vi "外观 1.vi"(0 "Data In":T5 caption="数据输入", 2 "Display State In":T3 caption="显示状态输入", 3 "Container State":T4 caption="容器状态") -> (6 "Data Out":T5 caption="数据输出", 7 "Display State Out":T3 caption="显示状态输出", 8 "Action":T2 caption="动作")   [LabVIEW 2016, in "曲线模型.xctl"]
uses:
  <vilib>/_xctls/Container State.ctl
  <vilib>/_xctls/Action.ctl
  <vilib>/_xctls/XControlSupport.lvlib
  <vilib>/Utility/config.llb/NI_LVConfig.lvlib
panel:
  in  "曲线模型":T1={"标液浓度1"=0.0, "样品1 F0"=0.0, "样品1 F1"=0.0, "测量吸光度1"=0.0, "样品1启用"=FALSE, "标液浓度2"=0.0, "样品2 F0"=0.0, "样品2 F1"=0.0, "测量吸光度2"=0.0, "样品2启用"=FALSE, "标液浓度3"=0.0, "样品3 F0"=0.0, "样品3 F1"=0.0, "测量吸光度3"=0.0, "样品3启用"=FALSE, "标液浓度4"=0.0, "样品4 F0"=0.0, "样品4 F1"=0.0, "测量吸光度4"=0.0, "样品4启用"=FALSE, "标液浓度5"=0.0, "样品5 F0"=0.0, "样品5 F1"=0.0, "测量吸光度5"=0.0, "样品5启用"=FALSE, "模型"=enum."线性", "method"=enum."最小二乘", "精度"=4.0, "XY图"=[], "拟合公式"="", "r^2"=0.0, "吸光值算法"=enum."对数"} {"r^2" format="%.7g"}
  # "标液浓度"
  # "F0"
  # "F1"
  # "吸光值显示"
  # "辅\n助\n计\n算\n区"
  # "样品一"
  # "样品二"
  # "样品三"
  # "样品四"
  # "样品五"
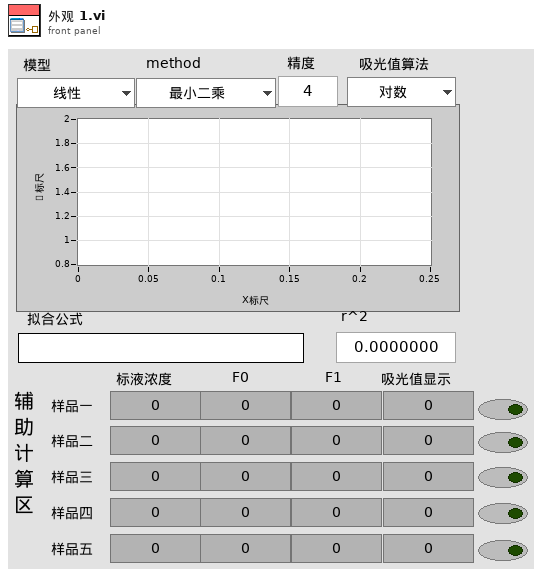
[diagram p1: front panel]
types:
  T1 = typedef "曲线模型.xctl/曲线模型外观.ctl" = cluster{"标液浓度1":dbl, "样品1 F0":dbl, "样品1 F1":dbl, "测量吸光度1":dbl, "样品1启用":bool, "标液浓度2":dbl, "样品2 F0":dbl, "样品2 F1":dbl, "测量吸光度2":dbl, "样品2启用":bool, "标液浓度3":dbl, "样品3 F0":dbl, "样品3 F1":dbl, "测量吸光度3":dbl, "样品3启用":bool, "标液浓度4":dbl, "样品4 F0":dbl, "样品4 F1":dbl, "测量吸光度4":dbl, "样品4启用":bool, "标液浓度5":dbl, "样品5 F0":dbl, "样品5 F1":dbl, "测量吸光度5":dbl, "样品5启用":bool, "模型":enum32{"线性", "多项式"}, "method":enum16{"最小二乘", "最小绝对残差", "Bisquare"}, "精度":dbl, "XY图":cluster{"X Values":dbl[], "Y Values":dbl[]}[], "拟合公式":string, "r^2":dbl, "吸光值算法":enum16{"对数", "减法"}}
  T2 = typedef "XControlSupport.lvlib/Action.ctl" = cluster{"Data Changed?":bool, "State Changed?":bool, "Action Name":string}
  T3 = typedef "曲线模型.xctl/状态 1.ctl" = cluster{"模型选择":cluster{"参数":u8, "测量模式":u8, "量程":u8}, "吸光值":cluster{"Value":dbl, "Value 2":dbl, "Value 3":dbl, "Value 4":dbl, "Value 5":dbl}, "浓度":cluster{"标液浓度1":dbl, "标液浓度2":dbl, "标液浓度3":dbl, "标液浓度4":dbl, "标液浓度5":dbl}}
  T4 = typedef "XControlSupport.lvlib/Container State.ctl" = cluster{"Indicator?":bool, "Run Mode?":bool, " Refnum":refnum<vi>}
  T5 = typedef "曲线模型.xctl/数据 1.ctl" = cluster{"X^2":dbl, "X":dbl, "B":dbl, "r^2":dbl}
  T6 = cluster{"曲线模型":T1, "Polynomial Coefficients":dbl[]}
  T7 = cluster{"Value":dbl, "Value 2":dbl, "Value 3":dbl, "Value 4":dbl, "Value 5":dbl}
  T8 = typedef "NI_LVConfig.lvlib/Config Data RefNum.ctl" = refnum<k1>
  T9 = cluster{"Polynomial Coefficients[0]":dbl, "Polynomial Coefficients[1]":dbl, "Polynomial Coefficients[2]":dbl, "Polynomial Coefficients[3]":dbl}
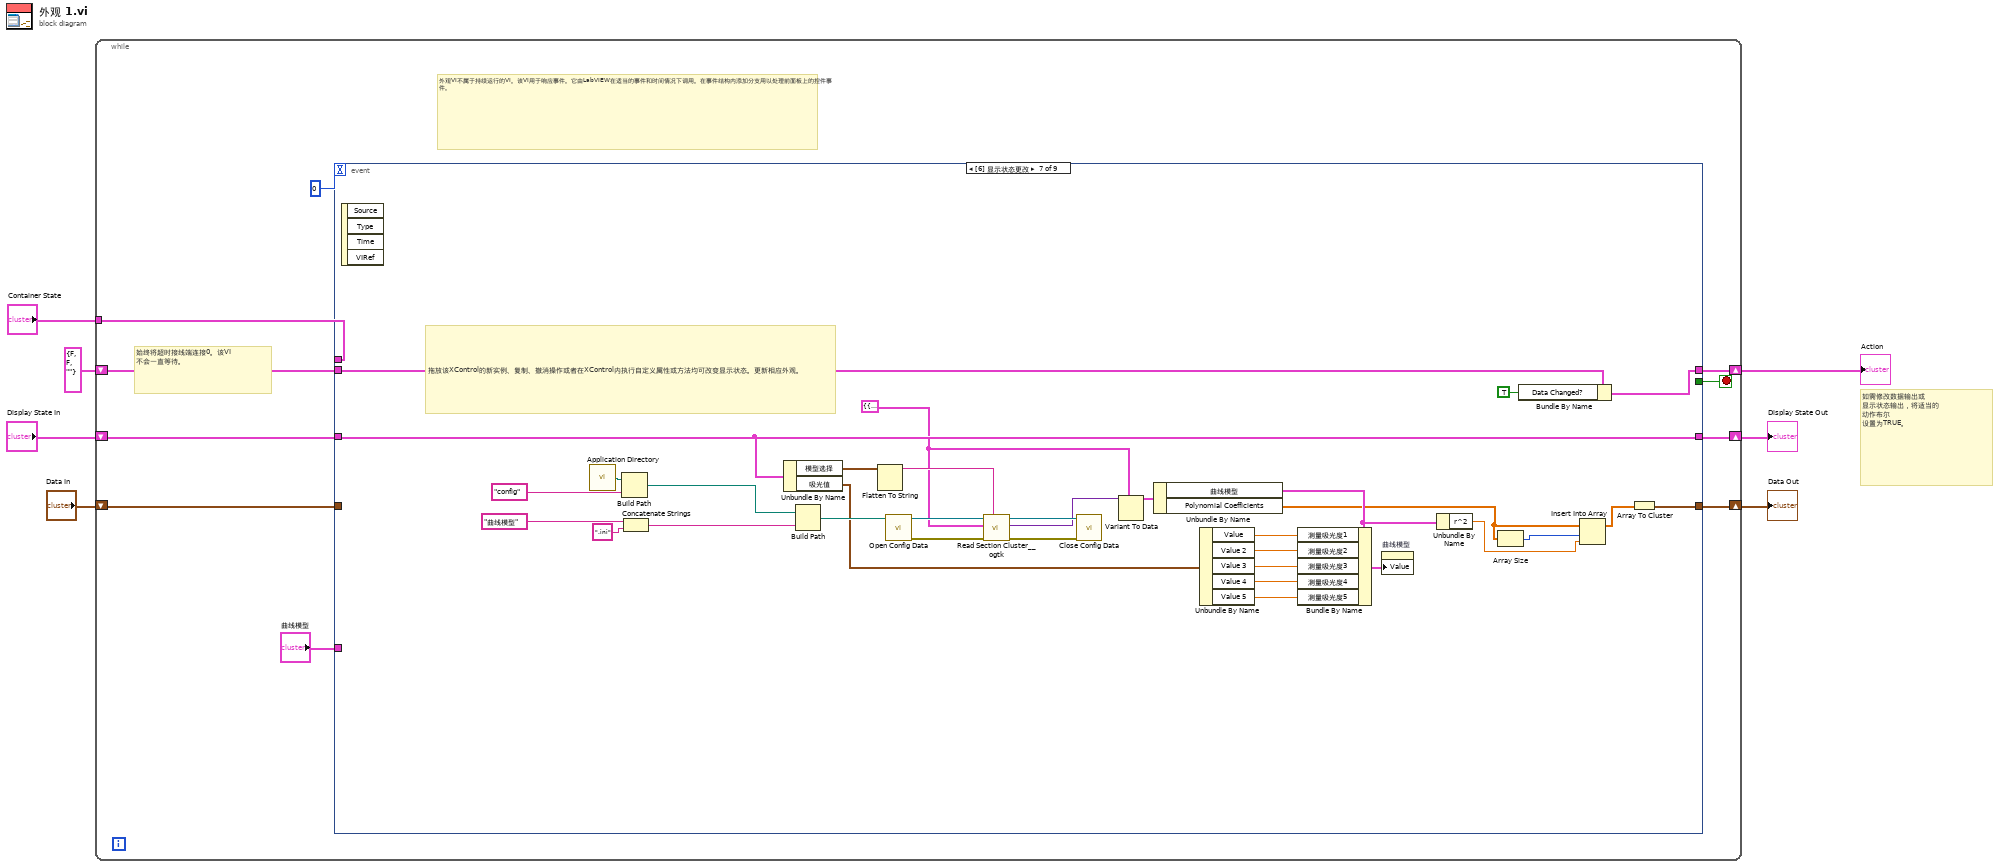
[diagram p0: block diagram]
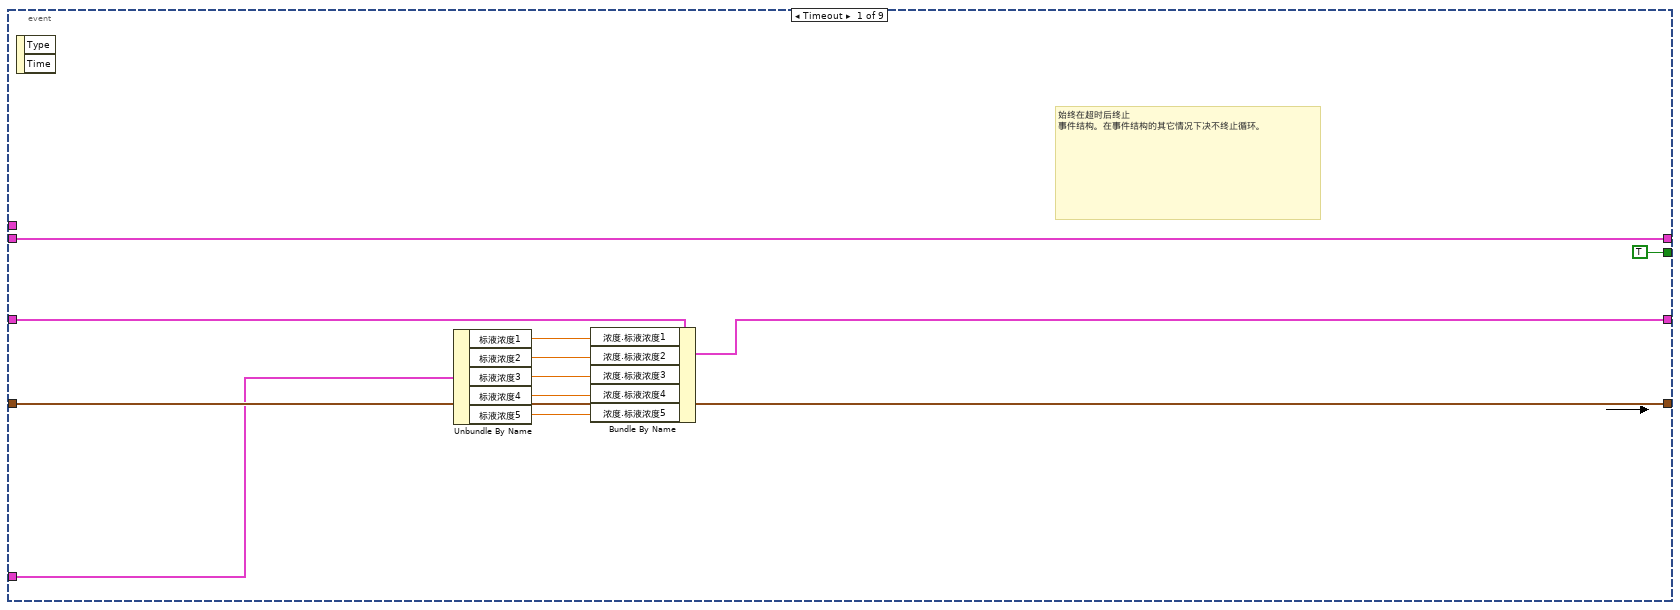
[diagram p2: hidden frame]
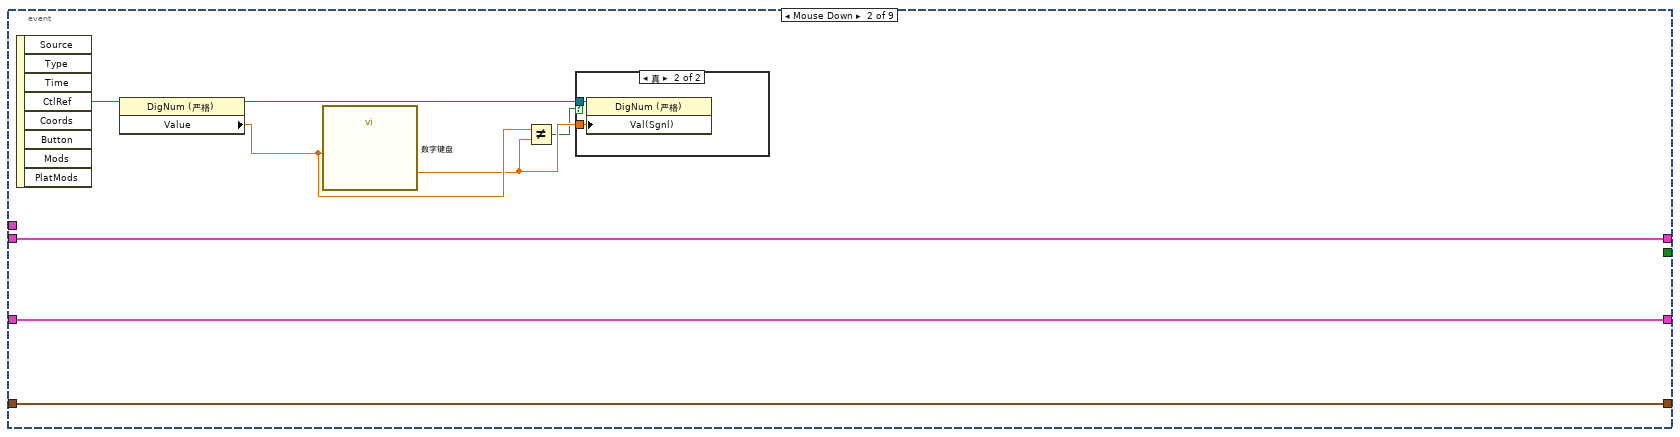
[diagram p3: hidden frame]
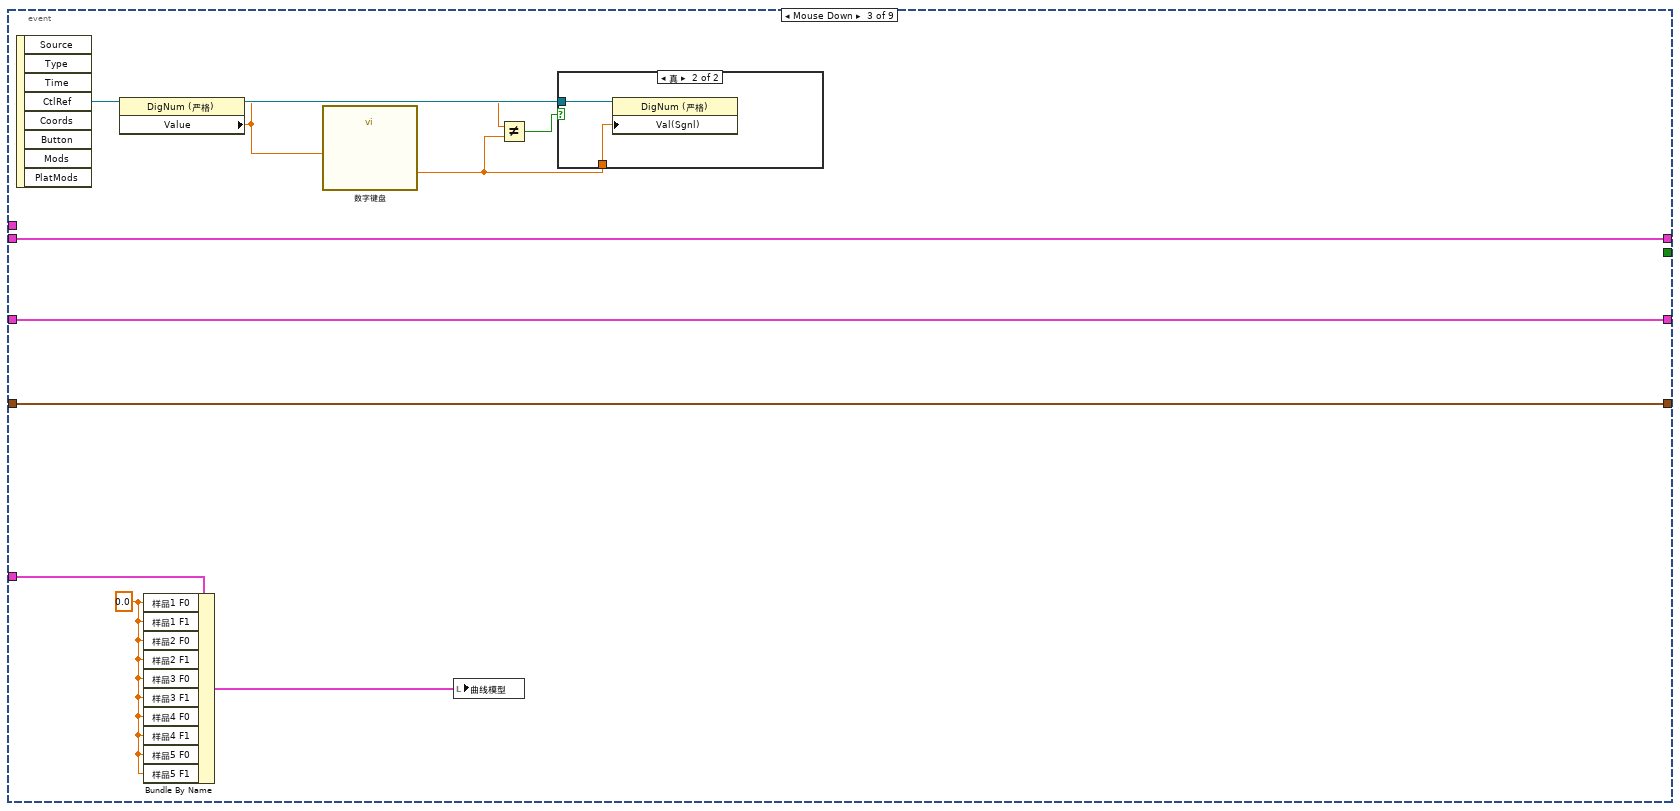
[diagram p5: hidden frame]
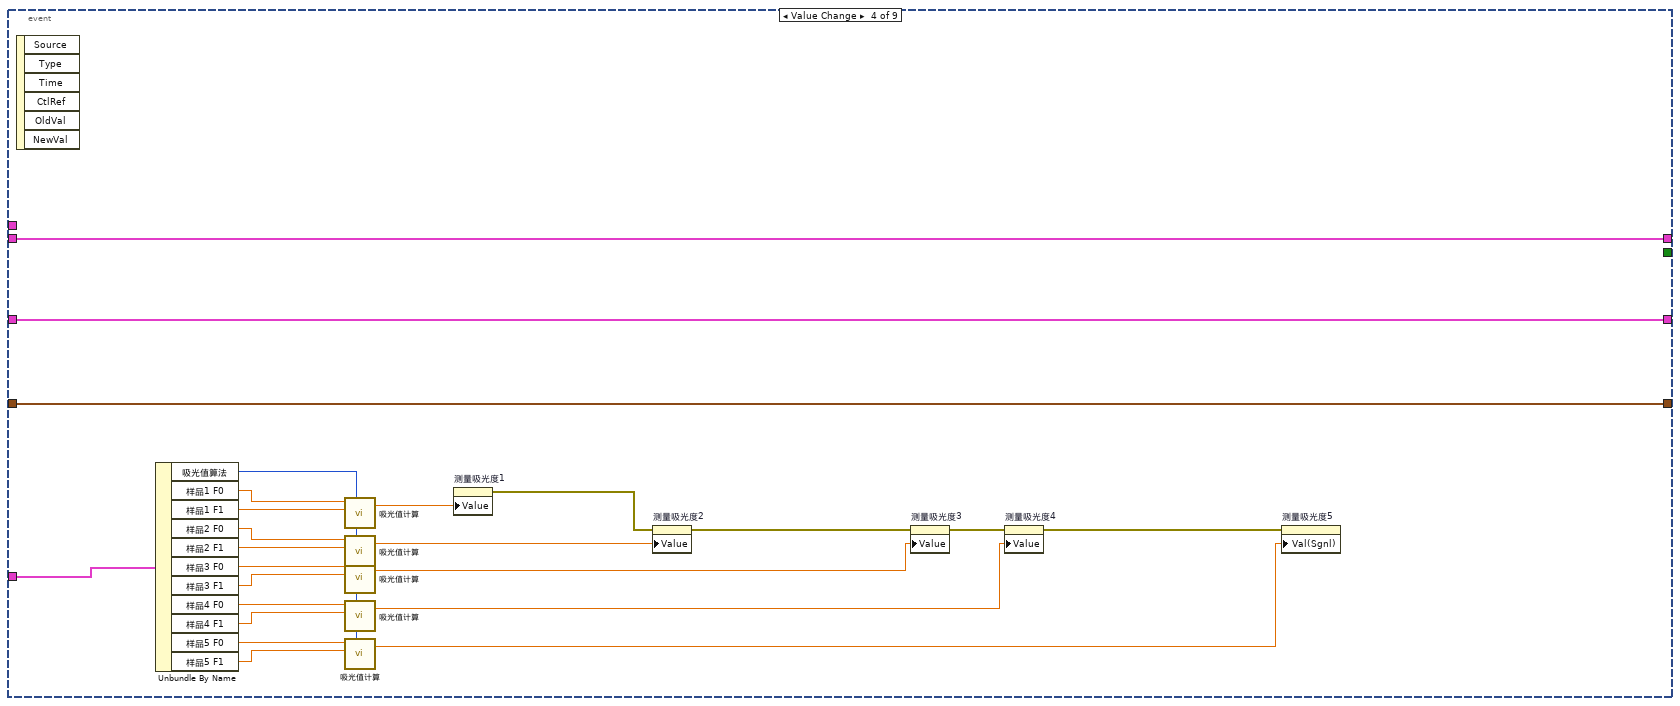
[diagram p7: hidden frame]
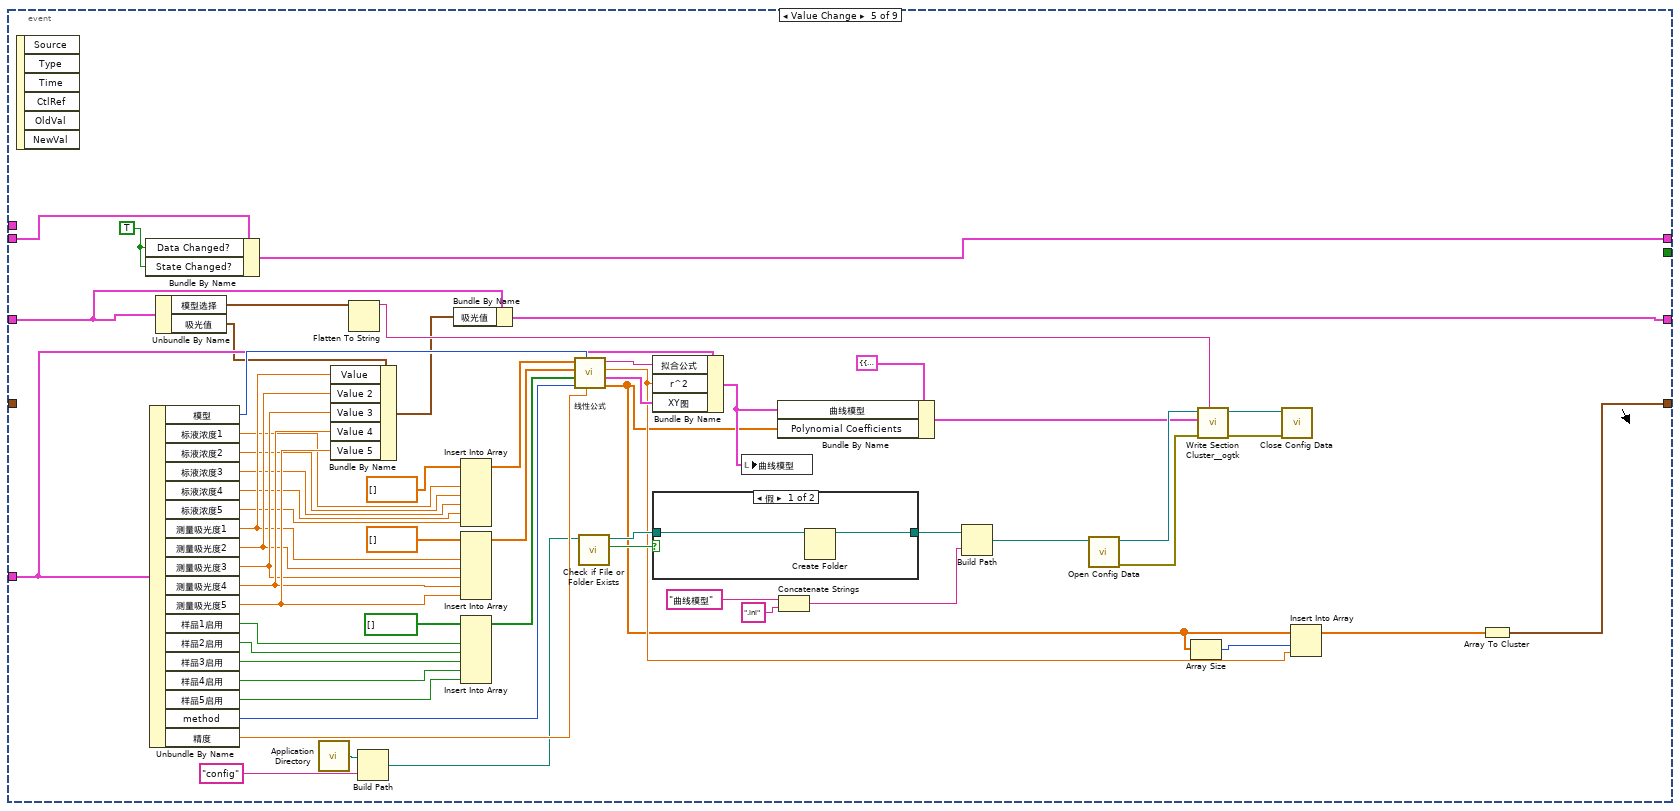
[diagram p8: hidden frame]
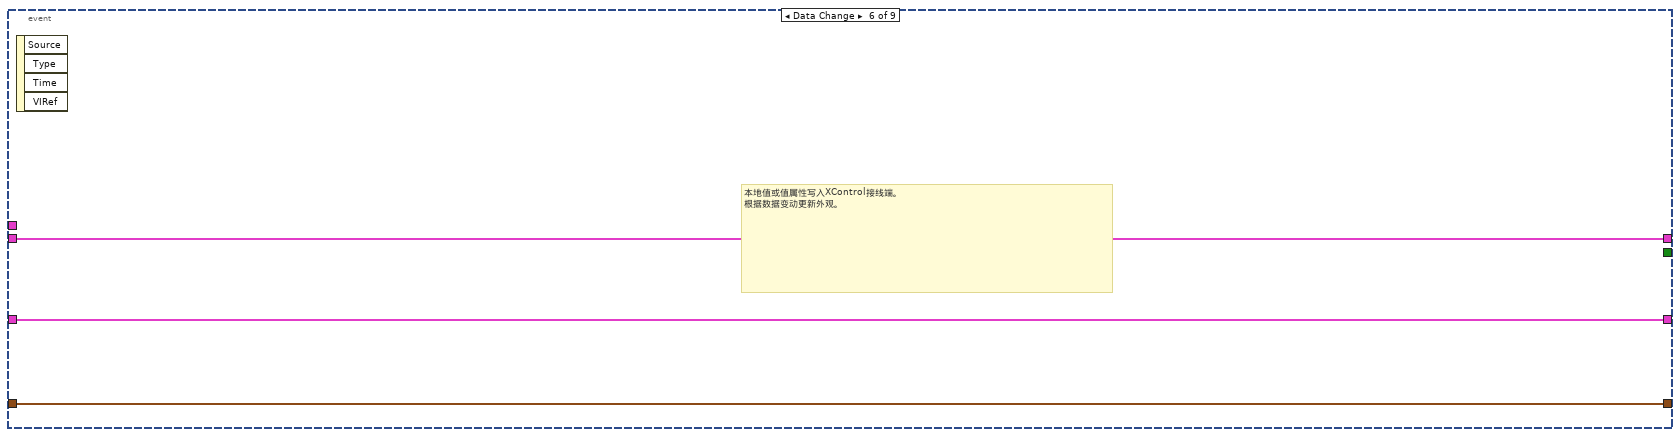
[diagram p10: hidden frame]
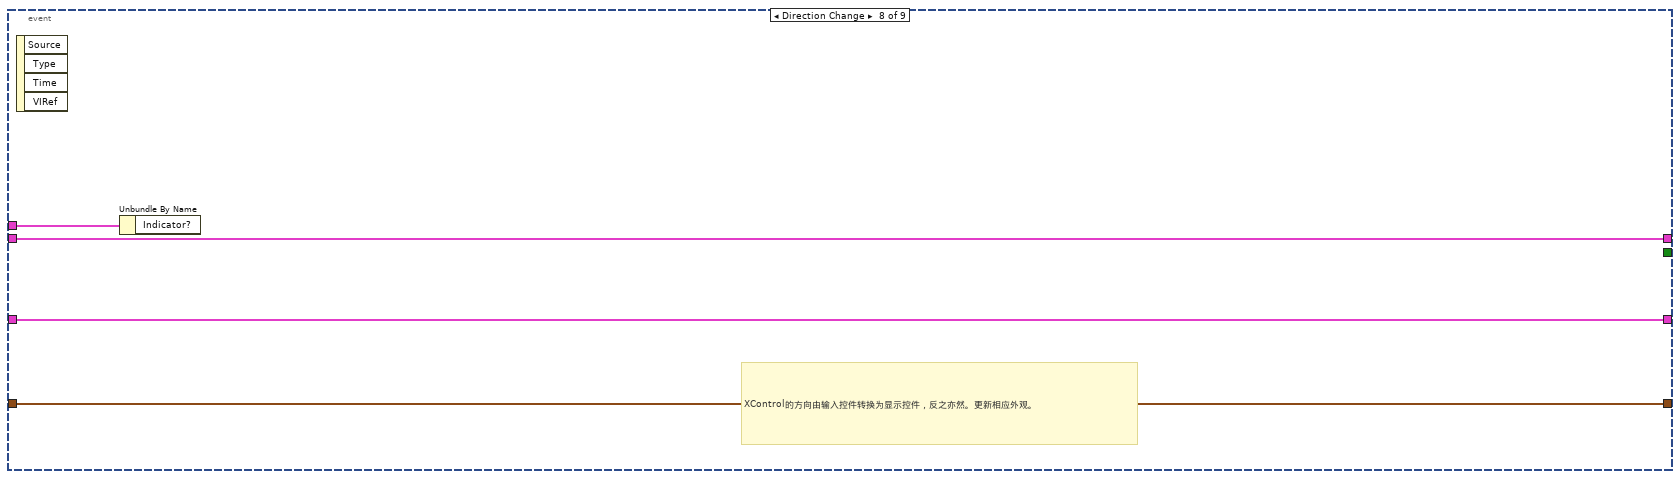
[diagram p11: hidden frame]
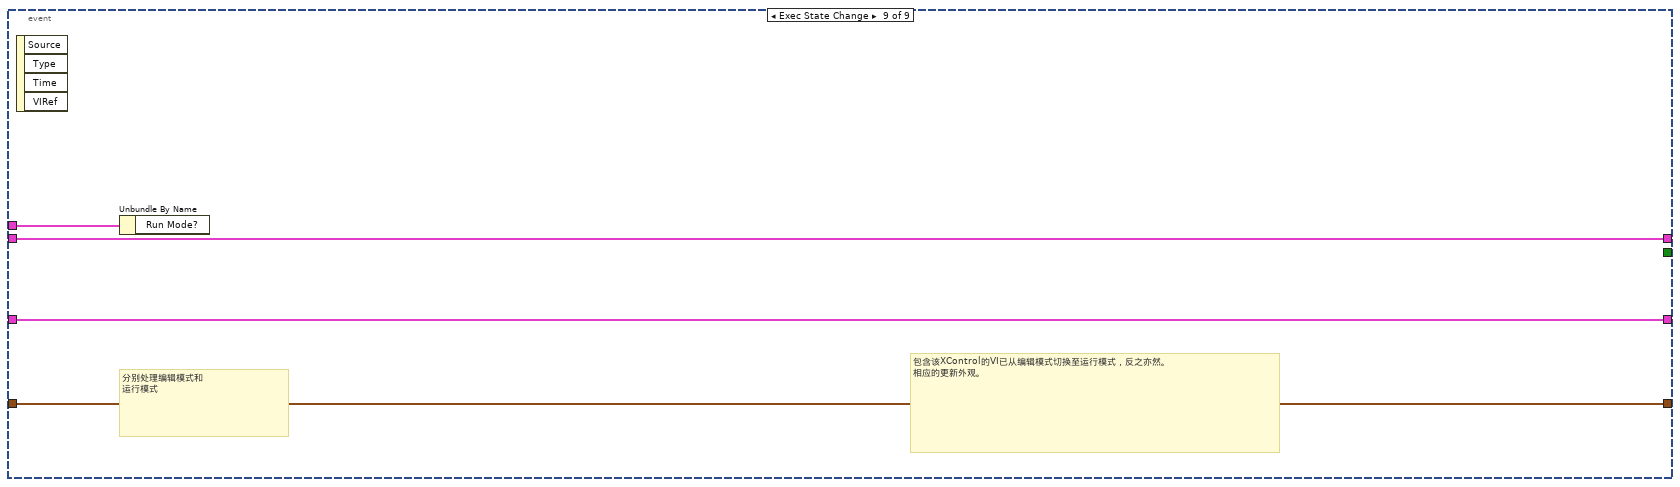
[diagram p12: hidden frame]
diagram:
  # "如需修改数据输出或\n显示状态输出，将适当的\n动作布尔\n设置为TRUE。"
  n1 = while {
    shift-right: [w16] -> w4
    shift-left: "Display State In" -> [w17]
    tunnel: "Container State" -> [w13]
    shift-right: [w11] -> w7
    shift-left: "Data In" -> [w12]
    shift-right: [w9] -> w2
    shift-left: T2 {"Data Changed?"=FALSE, "State Changed?"=FALSE, "Action Name"=""} ("Action") -> [w10]
    stop <- w15 stop-if-true
    # "外观VI不属于持续运行的VI。该VI用于响应事件。它由LabVIEW在适当的事件和时间情况下调用。在事件结构内添加分支用以处理前面板上的控件事件。"
    # "始终将超时接线端连接0。该VI\n不会一直等待。"
    n2 = event shown="[6] 显示状态更改" {
      selector: _ -> [_ _ _ _ _ _ _ _ _]
      dyn-events: _ -> [_ _ _ _ _ _ _ _ _]
      timeout: 0 -> [_ _ _ _ _ _ _ _ _]
      tunnel: w17 -> [w26 w32 w49 w75 w105 w137 w146 w175 w179]
      tunnel: [w24 w32 w49 w75 w93 w137 w146 w175 w179] -> w16
      tunnel: [TRUE _ _ _ _ _ _ _ _] -> w15
      tunnel: w13 -> [_ _ _ _ _ _ _ w176 w180]
      tunnel: w12 -> [w25 w36 w48 w74 _ w139 _ w174 w178]
      tunnel: [w25 w36 w48 w74 w116 w139 w157 w174 w178] -> w11
      tunnel: [w27 w35 w47 w73 w114 w138 w154 w173 w177] -> w9
      tunnel: w10 -> [w27 w35 w47 w73 w115 w138 w156 w173 w177]
      tunnel: "曲线模型" -> [w23 _ w44 w62 w119 _ _ _ _]
      event Timeout {
        # "始终在超时后终止\n事件结构。在事件结构的其它情况下决不终止循环。"
        n3 = event-data() -> ()  [unwired: 1 in, 2 out]
        n4 = Unbundle By Name(w23) -> ("标液浓度1"=w22:dbl, "标液浓度2"=w21:dbl, "标液浓度3"=w20:dbl, "标液浓度4"=w19:dbl, "标液浓度5"=w18:dbl)
        n5 = Bundle By Name(cluster=w26, "浓度.标液浓度1"=w22, "浓度.标液浓度2"=w21, "浓度.标液浓度3"=w20, "浓度.标液浓度4"=w19, "浓度.标液浓度5"=w18) -> (w24:T3)
      }
      event Mouse Down {
        n6 = event-data() -> ("CtlRef"=w34:refnum<vi>)  [unwired: 1 in, 7 out]
        n7 = property class="DigNum (严格)"(reference=w34) -> (reference out=w33:refnum<vi>, "Value"=w31:dbl)  [unwired: 1 in, 1 out]
        n8 = call "数字键盘.vi"("OldNumber"=w31) -> ("NewNumber"=w30:dbl)
        n9 = Not Equal?(x=w31, y=w30) -> (x != y?=w29:bool)
        n10 = case shown="真" w29 {
          tunnel: w33 -> [_ w38]
          tunnel: w30 -> [_ w37]
          frame False {
          }
          frame True {
            n11 = property class="DigNum (严格)"(reference=w38, "Val(Sgnl)"=w37) -> ()  [unwired: 1 in, 2 out]
          }
        }
      }
      event Mouse Down {
        w43 = 0.0 ("测量吸光度1")
        n12 = event-data() -> ("CtlRef"=w46:refnum<vi>)  [unwired: 1 in, 7 out]
        n13 = property class="DigNum (严格)"(reference=w46) -> (reference out=w45:refnum<vi>, "Value"=w41:dbl)  [unwired: 1 in, 1 out]
        n14 = Bundle By Name(cluster=w44, "样品1 F0"=w43, "样品1 F1"=w43, "样品2 F0"=w43, "样品2 F1"=w43, "样品3 F0"=w43, "样品3 F1"=w43, "样品4 F0"=w43, "样品4 F1"=w43, "样品5 F0"=w43, "样品5 F1"=w43) -> (w42:T1)
        n15 = call "数字键盘.vi"("OldNumber"=w41) -> ("NewNumber"=w40:dbl)
        n16 = local write "曲线模型"(w42) -> ()
        n17 = Not Equal?(x=w41, y=w40) -> (x != y?=w39:bool)
        n18 = case shown="真" w39 {
          tunnel: w45 -> [_ w51]
          tunnel: w40 -> [_ w50]
          frame False {
          }
          frame True {
            n19 = property class="DigNum (严格)"(reference=w51, "Val(Sgnl)"=w50) -> ()  [unwired: 1 in, 2 out]
          }
        }
      }
      event Value Change {
        n20 = event-data() -> ()  [unwired: 1 in, 6 out]
        n21 = Unbundle By Name(w62) -> ("吸光值算法"=w52:enum16{"对数", "减法"}, "样品1 F0"=w72:dbl, "样品1 F1"=w71:dbl, "样品2 F0"=w63:dbl, "样品2 F1"=w64:dbl, "样品3 F0"=w65:dbl, "样品3 F1"=w66:dbl, "样品4 F0"=w67:dbl, "样品4 F1"=w68:dbl, "样品5 F0"=w69:dbl, "样品5 F1"=w70:dbl)
        n22 = call "吸光值计算.vi"("吸光值算法"=w52, "F1"=w71, "F0"=w72) -> ("测量吸光度"=w57:dbl)  [unwired: 4 in]
        n23 = call "吸光值计算.vi"("吸光值算法"=w52, "F1"=w64, "F0"=w63) -> ("测量吸光度"=w56:dbl)  [unwired: 4 in]
        n24 = call "吸光值计算.vi"("吸光值算法"=w52, "F1"=w66, "F0"=w65) -> ("测量吸光度"=w55:dbl)  [unwired: 4 in]
        n25 = call "吸光值计算.vi"("吸光值算法"=w52, "F1"=w68, "F0"=w67) -> ("测量吸光度"=w54:dbl)  [unwired: 4 in]
        n26 = call "吸光值计算.vi"("吸光值算法"=w52, "F1"=w70, "F0"=w69) -> ("测量吸光度"=w53:dbl)  [unwired: 4 in]
        n27 = property on="测量吸光度1" class="DigNum (严格)"("Value"=w57) -> (error out=w61:errorcluster)  [unwired: 2 in, 1 out]
        n28 = property on="测量吸光度2" class="DigNum (严格)"(error in=w61, "Value"=w56) -> (error out=w60:errorcluster)  [unwired: 1 in, 1 out]
        n29 = property on="测量吸光度3" class="DigNum (严格)"(error in=w60, "Value"=w55) -> (error out=w59:errorcluster)  [unwired: 1 in, 1 out]
        n30 = property on="测量吸光度4" class="DigNum (严格)"(error in=w59, "Value"=w54) -> (error out=w58:errorcluster)  [unwired: 1 in, 1 out]
        n31 = property on="测量吸光度5" class="DigNum (严格)"(error in=w58, "Val(Sgnl)"=w53) -> ()  [unwired: 1 in, 2 out]
      }
      event Value Change {
        w76 = TRUE ("Data Changed?")
        n32 = event-data() -> ()  [unwired: 1 in, 6 out]
        n33 = Bundle By Name(cluster=w115, "Data Changed?"=w76, "State Changed?"=w76) -> (w114:T2)
        n34 = Unbundle By Name(w119) -> ("模型"=w133:enum32{"线性", "多项式"}, "标液浓度1"=w85:dbl, "标液浓度2"=w84:dbl, "标液浓度3"=w83:dbl, "标液浓度4"=w82:dbl, "标液浓度5"=w81:dbl, "测量吸光度1"=w86:dbl, "测量吸光度2"=w87:dbl, "测量吸光度3"=w88:dbl, "测量吸光度4"=w89:dbl, "测量吸光度5"=w90:dbl, "样品1启用"=w125:bool, "样品2启用"=w124:bool, "样品3启用"=w123:bool, "样品4启用"=w122:bool, "样品5启用"=w121:bool, "method"=w132:enum16{"最小二乘", "最小绝对残差", "Bisquare"}, "精度"=w131:dbl)
        n35 = Unbundle By Name(w105) -> ("模型选择"=w104:cluster{"参数":u8, "测量模式":u8, "量程":u8}, "吸光值"=w91:T7)
        n36 = call <vilib>:"Application Directory.vi"() -> ("Application Directory"=w113:path)
        n37 = Bundle By Name(cluster=w91, "Value"=w86, "Value 2"=w87, "Value 3"=w88, "Value 4"=w89, "Value 5"=w90) -> (w92:T7)
        n38 = Flatten To String(anything=w104) -> (data string=w103:string)  [unwired: 3 in, 2 out]
        n39 = Build Path(base path=w113, name or relative path="config" ("名称或相对路径")) -> (appended path=w111:path)
        n40 = Bundle By Name(cluster=w105, "吸光值"=w92) -> (w93:T3)
        n41 = Insert Into Array(array=dbl[] [] ("标液浓度"), new element #1=w85, new element #2=w84, new element #3=w83, new element #4=w82, new element #5=w81) -> (w129:dbl[])  [unwired: 1 in]
        n42 = Insert Into Array(array=dbl[] [] ("标液浓度"), new element #1=w86, new element #2=w87, new element #3=w88, new element #4=w89, new element #5=w90) -> (w127:dbl[])  [unwired: 1 in]
        n43 = Insert Into Array(array=bool[] [] ("启用"), new element #1=w125, new element #2=w124, new element #3=w123, new element #4=w122, new element #5=w121) -> (w120:bool[])  [unwired: 1 in]
        n44 = call "线性公式.vi"("精度"=w131, "模型"=w133, "method"=w132, "启用"=w120, "监测浓度"=w127, "标液浓度"=w129) -> ("Polynomial Coefficients"=w78:dbl[], "XY图"=w117:cluster{"X Values":dbl[], "Y Values":dbl[]}[], "r^2"=w79:dbl, "拟合方程"=w118:string)  [unwired: 2 in]
        n45 = call <vilib>:"Check if File or Folder Exists.vi"("path"=w111) -> ("file or folder exists?"=w110:bool, "dup path"=w109:path)  [unwired: 8 in, 1 out]
        n46 = Bundle By Name(cluster=w119, "拟合公式"=w118, "r^2"=w79, "XY图"=w117) -> (w95:T1)
        n47 = case shown="假" w110 {
          tunnel: w109 -> [w135 w136]
          tunnel: [w134 w136] -> w106
          frame False {
            n48 = Create Folder(path (use dialog)=w135) -> (created path=w134:path)  [unwired: 2 in, 2 out]
          }
          frame True {
          }
        }
        n49 = local write "曲线模型"(w95) -> ()
        n50 = Bundle By Name(cluster=T6 {"曲线模型"={"标液浓度1"=0.0, "样品1 F0"=0.0, "样品1 F1"=0.0, "测量吸光度1"=0.0, "样品1启用"=FALSE, "标液浓度2"=0.0, "样品2 F0"=0.0, "样品2 F1"=0.0, "测量吸光度2"=0.0, "样品2启用"=FALSE, "标液浓度3"=0.0, "样品3 F0"=0.0, "样品3 F1"=0.0, "测量吸光度3"=0.0, "样品3启用"=FALSE, "标液浓度4"=0.0, "样品4 F0"=0.0, "样品4 F1"=0.0, "测量吸光度4"=0.0, "样品4启用"=FALSE, "标液浓度5"=0.0, "样品5 F0"=0.0, "样品5 F1"=0.0, "测量吸光度5"=0.0, "样品5启用"=FALSE, "模型"=enum."线性", "method"=enum."最小二乘", "精度"=4.0, "XY图"=[], "拟合公式"="", "r^2"=0.0, "吸光值算法"=enum."对数"}, "Polynomial Coefficients"=[]} ("输出簇"), "曲线模型"=w95, "Polynomial Coefficients"=w78) -> (w94:T6)
        n51 = Concatenate Strings("曲线模型" ("字符串"), ".ini" ("字符串")) -> (w108:string)
        n52 = Build Path(base path=w106, name or relative path=w108) -> (appended path=w97:path)
        n53 = call <vilib>:"Open Config Data.vi"("configuration file path"=w97) -> ("error out"=w100:errorcluster, "refnum"=w101:T8)  [unwired: 8 in, 1 out]
        n54 = Array Size(array=w78) -> (size(s)=w77:i32)
        n55 = call <userlib>:"Write Section Cluster__ogtk.vi"("section (optional)"=w103, "error in (no error)"=w100, "Section Formatted Cluster"=w94, "refnum"=w101) -> ("error out"=w98:errorcluster, "dup refnum"=w99:T8)  [unwired: 6 in]
        n56 = call <vilib>:"Close Config Data.vi"("error in (no error)"=w98, "refnum"=w99) -> ()  [unwired: 8 in, 2 out]
        n57 = Insert Into Array(array=w78, index=w77, new element=w79) -> (w80:dbl[])
        n58 = Array To Cluster(array=w80) -> (cluster=w116:T9)
      }
      event Data Change {
        # "本地值或值属性写入XControl接线端。\n根据数据变动更新外观。"
        n59 = event-data() -> ()  [unwired: 1 in, 4 out]
      }
      event Display State Change {
        w140 = T6 {"曲线模型"={"标液浓度1"=0.0, "样品1 F0"=0.0, "样品1 F1"=0.0, "测量吸光度1"=0.0, "样品1启用"=FALSE, "标液浓度2"=0.0, "样品2 F0"=0.0, "样品2 F1"=0.0, "测量吸光度2"=0.0, "样品2启用"=FALSE, "标液浓度3"=0.0, "样品3 F0"=0.0, "样品3 F1"=0.0, "测量吸光度3"=0.0, "样品3启用"=FALSE, "标液浓度4"=0.0, "样品4 F0"=0.0, "样品4 F1"=0.0, "测量吸光度4"=0.0, "样品4启用"=FALSE, "标液浓度5"=0.0, "样品5 F0"=0.0, "样品5 F1"=0.0, "测量吸光度5"=0.0, "样品5启用"=FALSE, "模型"=enum."线性", "method"=enum."最小二乘", "精度"=4.0, "XY图"=[], "拟合公式"="", "r^2"=0.0, "吸光值算法"=enum."对数"}, "Polynomial Coefficients"=[]} ("输出簇")
        # "拖放该XControl的新实例、复制、撤消操作或者在XControl内执行自定义属性或方法均可改变显示状态。更新相应外观。"
        n60 = event-data() -> ()  [unwired: 1 in, 4 out]
        n61 = call <vilib>:"Application Directory.vi"() -> ("Application Directory"=w167:path)
        n62 = Build Path(base path=w167, name or relative path="config" ("名称或相对路径")) -> (appended path=w165:path)
        n63 = Concatenate Strings("曲线模型" ("字符串"), ".ini" ("字符串")) -> (w163:string)
        n64 = Unbundle By Name(w146) -> ("模型选择"=w161:cluster{"参数":u8, "测量模式":u8, "量程":u8}, "吸光值"=w153:T7)
        n65 = Build Path(base path=w165, name or relative path=w163) -> (appended path=w168:path)
        n66 = Flatten To String(anything=w161) -> (data string=w160:string)  [unwired: 3 in, 2 out]
        n67 = call <vilib>:"Open Config Data.vi"("configuration file path"=w168) -> ("error out"=w171:errorcluster, "refnum"=w172:T8)  [unwired: 8 in, 1 out]
        n68 = call <userlib>:"Read Section Cluster__ogtk.vi"("section (optional)"=w160, "error in (no error)"=w171, "Section Formatted Cluster Type"=w140, "refnum"=w172) -> ("error out"=w169:errorcluster, "Section Formatted Cluster"=w162:variant, "dup refnum"=w170:T8)  [unwired: 3 in, 2 out]
        n69 = call <vilib>:"Close Config Data.vi"("error in (no error)"=w169, "refnum"=w170) -> ()  [unwired: 8 in, 2 out]
        n70 = Variant To Data(type=w140, Variant=w162) -> (data=w158:T6)  [unwired: 1 in, 1 out]
        n71 = Unbundle By Name(w158) -> ("曲线模型"=w145:T1, "Polynomial Coefficients"=w143:dbl[])
        n72 = Unbundle By Name(w153) -> ("Value"=w152:dbl, "Value 2"=w151:dbl, "Value 3"=w150:dbl, "Value 4"=w149:dbl, "Value 5"=w148:dbl)
        n73 = Bundle By Name(cluster=w145, "测量吸光度1"=w152, "测量吸光度2"=w151, "测量吸光度3"=w150, "测量吸光度4"=w149, "测量吸光度5"=w148) -> (w147:T1)
        n74 = property on="曲线模型" class="Clust (严格)"("Value"=w147) -> ()  [unwired: 2 in, 2 out]
        n75 = Unbundle By Name(w145) -> ("r^2"=w142:dbl)
        n76 = Array Size(array=w143) -> (size(s)=w144:i32)
        n77 = Bundle By Name(cluster=w156, "Data Changed?"=TRUE) -> (w154:T2)
        n78 = Insert Into Array(array=w143, index=w144, new element=w142) -> (w141:dbl[])
        n79 = Array To Cluster(array=w141) -> (cluster=w157:T9)
      }
      event Direction Change {
        # "XControl的方向由输入控件转换为显示控件，反之亦然。更新相应外观。"
        n80 = event-data() -> ()  [unwired: 1 in, 4 out]
        n81 = Unbundle By Name(w176) -> ()  [unwired: 1 out]
      }
      event Exec State Change {
        # "包含该XControl的VI已从编辑模式切换至运行模式，反之亦然。\n相应的更新外观。"
        # "分别处理编辑模式和\n运行模式"
        n82 = event-data() -> ()  [unwired: 1 in, 4 out]
        n83 = Unbundle By Name(w180) -> ()  [unwired: 1 out]
      }
    }
  }
  "Display State Out" <- w4
  "Data Out" <- w7
  "Action" <- w2
